vi "initialize hardware.vi"(7 "Reset (False)":bool, 8 "error in (no error)":errorcluster, 9 "devport":string, 10 "Settings":T1={"devport"="", "Position"={"Axis 1"={"Value"=0.0, "Min"=0.0, "Max"=0.0, "StepSize"=0.0, "Tolerance"=0.0, "ValueActual"=0.0}, "Axis 2"={"Value"=0.0, "Min"=0.0, "Max"=0.0, "StepSize"=0.0, "Tolerance"=0.0, "ValueActual"=0.0}, "Axis 3"={"Value"=0.0, "Min"=0.0, "Max"=0.0, "StepSize"=0.0, "Tolerance"=0.0, "ValueActual"=0.0}}, "Power"={"Axis 1"=enum."off", "Axis 2"=enum."off", "Axis 3"=enum."off"}, "Status"={"Axis 1"=enum."Not referenced", "Axis 2"=enum."Not referenced", "Axis 3"=enum."Not referenced"}, "Backlash"={"Axis 1"={"Value"=0.0, "Min"=0.0, "Max"=0.0, "StepSize"=0.0, "Tolerance"=0.0, "ValueActual"=0.0}, "Axis 2"={"Value"=0.0, "Min"=0.0, "Max"=0.0, "StepSize"=0.0, "Tolerance"=0.0, "ValueActual"=0.0}, "Axis 3"={"Value"=0.0, "Min"=0.0, "Max"=0.0, "StepSize"=0.0, "Tolerance"=0.0, "ValueActual"=0.0}}, "Home"={"Axis 1"={"Value"=0.0, "Min"=0.0, "Max"=0.0, "StepSize"=0.0, "Tolerance"=0.0, "ValueActual"=0.0}, "Axis 2"={"Value"=0.0, "Min"=0.0, "Max"=0.0, "StepSize"=0.0, "Tolerance"=0.0, "ValueActual"=0.0}, "Axis 3"={"Value"=0.0, "Min"=0.0, "Max"=0.0, "StepSize"=0.0, "Tolerance"=0.0, "ValueActual"=0.0}}, "MoveToHardLimit"={"Axis 1"=enum."pos", "Axis 2"=enum."pos", "Axis 3"=enum."pos"}, "relativeMove"={"Axis 1neg"=enum."off", "Axis 2neg"=enum."off", "Axis 3neg"=enum."off", "Axis 1pos"=enum."off", "Axis 2pos"=enum."off", "Axis 3pos"=enum."off"}, "stepsize"={"Value"=0.0, "Min"=0.0, "Max"=0.0, "StepSize"=0.0, "Tolerance"=0.0, "ValueActual"=0.0}, "automotoroff"=enum."off", "ResetBeforeMove"=enum."off", "Enable"={"Axis 1"=enum."on", "Axis 2"=enum."on", "Axis 3"=enum."on"}}, 11 "ESP301 in":refnum<class "ESP301.lvclass">) -> (0 "error out":errorcluster, 2 "VISA resource name out":refnum<visa-resource-name>, 3 "ESP301 out":refnum<class "ESP301.lvclass">)   [LabVIEW 2020, in "ESP301.lvclass"]
uses:
  ESP301.lvclass
  ESP301/SettingsTypdef.ctl
  OnOffTypeDef.ctl
  status_TypDef.ctl
  Hardware limit.ctl
  ESP301.lvclass/ESP301.ctl
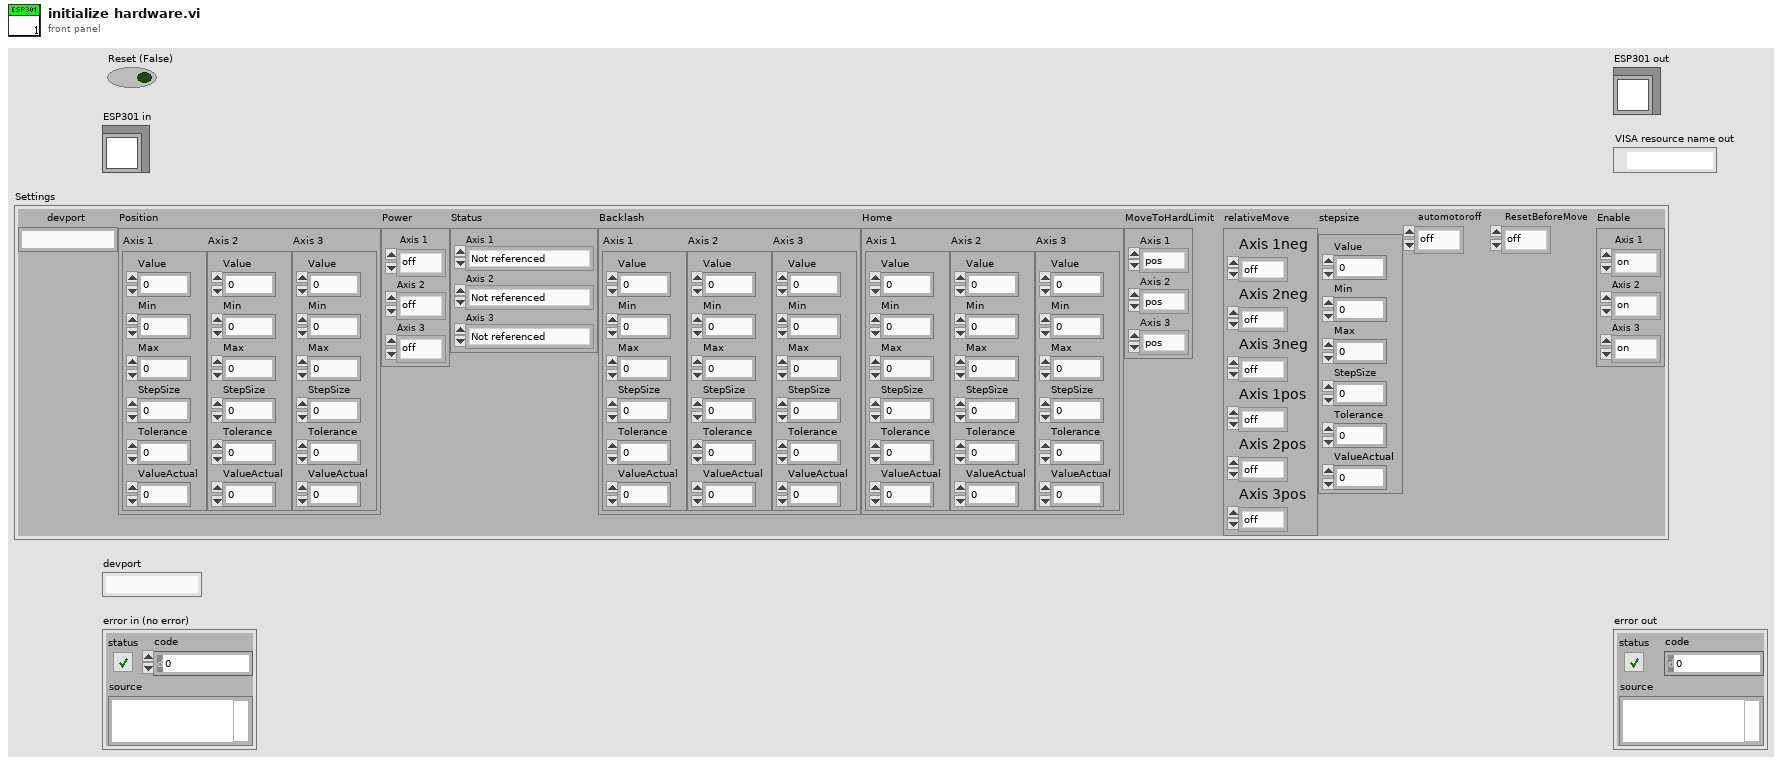
[diagram p1: front panel]
types:
  T1 = typedef "ESP301.lvclass/SettingsTypdef.ctl" = cluster{"devport":string, "Position":cluster{"Axis 1":cluster{"Value":dbl, "Min":dbl, "Max":dbl, "StepSize":dbl, "Tolerance":dbl, "ValueActual":dbl}, "Axis 2":cluster{"Value":dbl, "Min":dbl, "Max":dbl, "StepSize":dbl, "Tolerance":dbl, "ValueActual":dbl}, "Axis 3":cluster{"Value":dbl, "Min":dbl, "Max":dbl, "StepSize":dbl, "Tolerance":dbl, "ValueActual":dbl}}, "Power":cluster{"Axis 1":T2, "Axis 2":T2, "Axis 3":T2}, "Status":cluster{"Axis 1":T3, "Axis 2":T3, "Axis 3":T3}, "Backlash":cluster{"Axis 1":cluster{"Value":dbl, "Min":dbl, "Max":dbl, "StepSize":dbl, "Tolerance":dbl, "ValueActual":dbl}, "Axis 2":cluster{"Value":dbl, "Min":dbl, "Max":dbl, "StepSize":dbl, "Tolerance":dbl, "ValueActual":dbl}, "Axis 3":cluster{"Value":dbl, "Min":dbl, "Max":dbl, "StepSize":dbl, "Tolerance":dbl, "ValueActual":dbl}}, "Home":cluster{"Axis 1":cluster{"Value":dbl, "Min":dbl, "Max":dbl, "StepSize":dbl, "Tolerance":dbl, "ValueActual":dbl}, "Axis 2":cluster{"Value":dbl, "Min":dbl, "Max":dbl, "StepSize":dbl, "Tolerance":dbl, "ValueActual":dbl}, "Axis 3":cluster{"Value":dbl, "Min":dbl, "Max":dbl, "StepSize":dbl, "Tolerance":dbl, "ValueActual":dbl}}, "MoveToHardLimit":cluster{"Axis 1":T4, "Axis 2":T4, "Axis 3":T4}, "relativeMove":cluster{"Axis 1neg":T2, "Axis 2neg":T2, "Axis 3neg":T2, "Axis 1pos":T2, "Axis 2pos":T2, "Axis 3pos":T2}, "stepsize":cluster{"Value":dbl, "Min":dbl, "Max":dbl, "StepSize":dbl, "Tolerance":dbl, "ValueActual":dbl}, "automotoroff":T2, "ResetBeforeMove":T2, "Enable":cluster{"Axis 1":T2, "Axis 2":T2, "Axis 3":T2}}
  T2 = typedef "OnOffTypeDef.ctl" = enum16{"off", "on"}
  T3 = typedef "status_TypDef.ctl" = enum16{"Not referenced", "Homing", "Moving", "Ready"}
  T4 = typedef "Hardware limit.ctl" = enum16{"pos", "neg"}
  T5 = cluster{"Axis 1":cluster{"Value":dbl, "Min":dbl, "Max":dbl, "StepSize":dbl, "Tolerance":dbl, "ValueActual":dbl}, "Axis 2":cluster{"Value":dbl, "Min":dbl, "Max":dbl, "StepSize":dbl, "Tolerance":dbl, "ValueActual":dbl}, "Axis 3":cluster{"Value":dbl, "Min":dbl, "Max":dbl, "StepSize":dbl, "Tolerance":dbl, "ValueActual":dbl}}
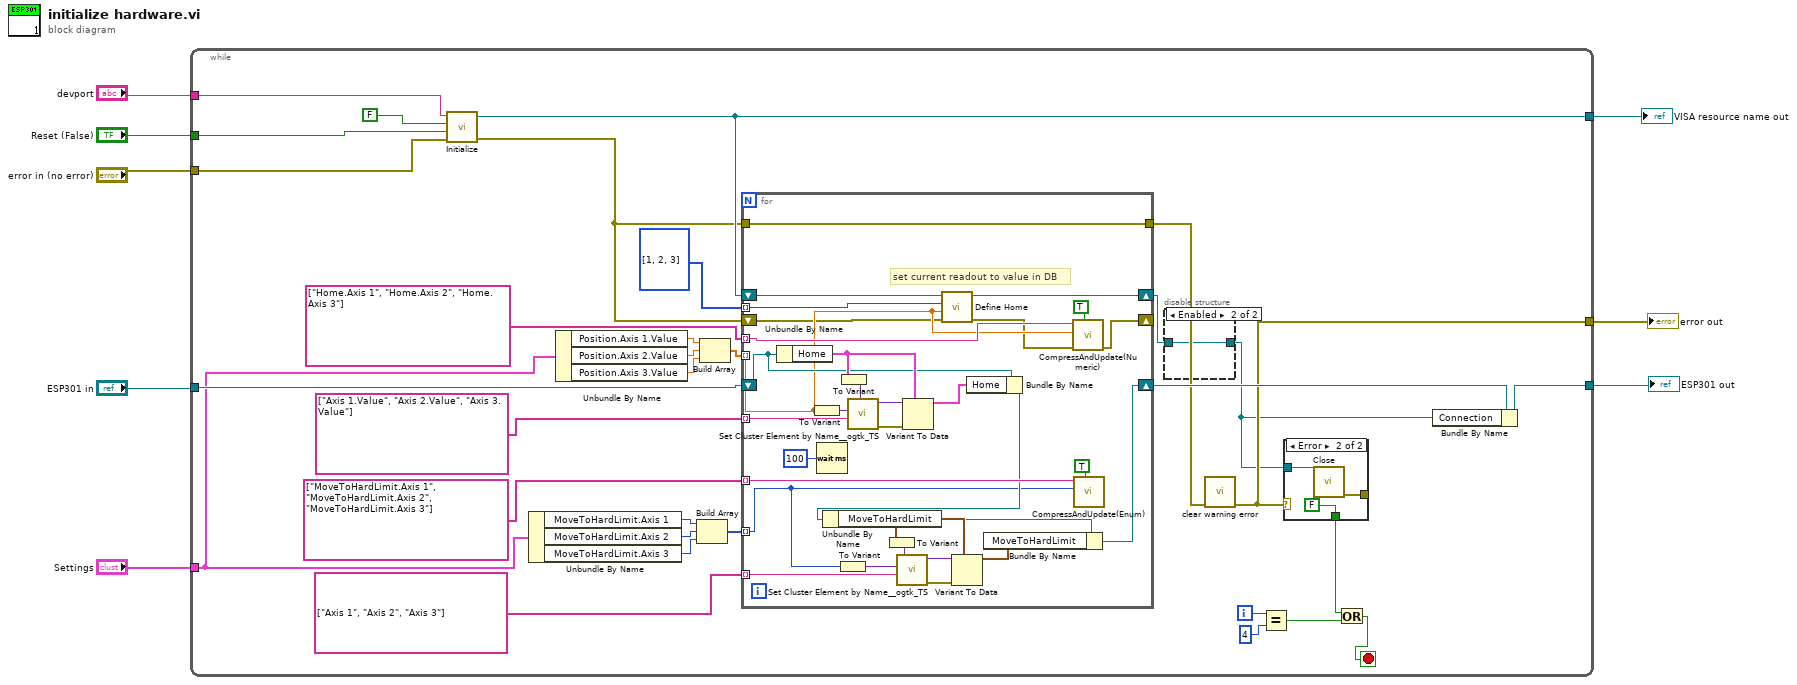
[diagram p0: block diagram]
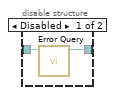
[diagram p2: hidden frame]
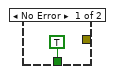
[diagram p3: hidden frame]
diagram:
  n1 = while {
    tunnel: "error in (no error)" -> [w13]
    tunnel: "devport" -> [w16]
    tunnel: "ESP301 in" -> [w35]
    tunnel: [w10] -> w4
    tunnel: [w15] -> w5
    tunnel: "Settings" -> [w24]
    tunnel: [w19] -> w7
    tunnel: "Reset (False)" -> [w11]
    i -> [w23]
    stop <- w20 stop-if-true
    n2 = call "Initialize.vi"("VISA resource name"=w16, "ID Query (True)"=FALSE, "Reset (False)"=w11, "error in (no error)"=w13) -> ("VISA resource name out"=w15:refnum<visa-resource-name>, "error out"=w14:errorcluster)  [unwired: 5 in]
    n3 = Unbundle By Name(w24) -> ("MoveToHardLimit.Axis 1"=w27:T4, "MoveToHardLimit.Axis 2"=w28:T4, "MoveToHardLimit.Axis 3"=w29:T4)
    n4 = Unbundle By Name(w24) -> ("Position.Axis 1.Value"=w39:dbl, "Position.Axis 2.Value"=w38:dbl, "Position.Axis 3.Value"=w37:dbl)
    n5 = Build Array(w27, w28, w29) -> (w26:T4[])
    n6 = Build Array(w39, w38, w37) -> (w36:dbl[])
    n7 = for {
      shift-right: [w69] -> w31
      shift-left: w15 -> [w70]
      tunnel: i32[] [1, 2, 3] -> [w68] mode=indexing
      tunnel: w36 -> [w67] mode=indexing
      shift-right: [w56] -> w34
      shift-left: w35 -> [w74]
      tunnel: string[] ["Axis 1.Value", "Axis 2.Value", "Axis 3.Value"] ("set following Variables (empty = all avriables)") -> [w73] mode=indexing
      tunnel: string[] ["Home.Axis 1", "Home.Axis 2", "Home.Axis 3"] ("set following Variables (empty = all avriables)") -> [w71] mode=indexing
      shift-right: [w64] -> _
      shift-left: w14 -> [w66]
      tunnel: string[] ["MoveToHardLimit.Axis 1", "MoveToHardLimit.Axis 2", "MoveToHardLimit.Axis 3"] ("set following Variables (empty = all avriables)") -> [w62] mode=indexing
      tunnel: w26 -> [w55] mode=indexing
      tunnel: string[] ["Axis 1", "Axis 2", "Axis 3"] ("set following Variables (empty = all avriables)") -> [w54] mode=indexing
      tunnel: w14 -> [w52]
      tunnel: [w52] -> w17
      # "set current readout to value in DB"
      n8 = Unbundle By Name(w74) -> ("Home"=w77:T5)
      n9 = To Variant(anything=w67) -> (Variant=w49:variant)
      n10 = Wait (ms)(milliseconds to wait=u32 100) -> ()  [unwired: 1 out]
      n11 = To Variant(anything=w55) -> (Variant=w50:variant)
      n12 = To Variant(anything=w77) -> (Variant=w48:variant)
      n13 = call "Set Cluster Element by Name__ogtk_TS.vi"("Element Name (\"\": New Element Data Name)"=w73, "New Element Value"=w49, "Cluster"=w48) -> ("error out"=w75:errorcluster, "VCluster out"=w76:variant)  [unwired: 6 in, 1 out]
      n14 = Variant To Data(error in=w75, type=w77, Variant=w76) -> (data=w78:T5)  [unwired: 1 out]
      n15 = call "Define Home.vi"("error in (no error)"=w66, "Home Position (0 units)"=w67, "Axis (1)"=w68, "VISA resource name"=w70) -> ("error out"=w65:errorcluster, "VISA resource name out"=w69:refnum<visa-resource-name>)  [unwired: 2 in]
      n16 = Bundle By Name(cluster=w74, "Home"=w78) -> (w57:refnum<class "ESP301.lvclass">)
      n17 = Unbundle By Name(w57) -> ("MoveToHardLimit"=w59:cluster{"Axis 1":T4, "Axis 2":T4, "Axis 3":T4})
      n18 = To Variant(anything=w59) -> (Variant=w51:variant)
      n19 = call "Set Cluster Element by Name__ogtk_TS.vi"("Element Name (\"\": New Element Data Name)"=w54, "New Element Value"=w50, "Cluster"=w51) -> ("error out"=w61:errorcluster, "VCluster out"=w60:variant)  [unwired: 6 in, 1 out]
      n20 = Variant To Data(error in=w61, type=w59, Variant=w60) -> (data=w58:cluster{"Axis 1":T4, "Axis 2":T4, "Axis 3":T4})  [unwired: 1 out]
      n21 = Bundle By Name(cluster=w57, "MoveToHardLimit"=w58) -> (w56:refnum<class "ESP301.lvclass">)
      n22 = call "CompressAndUpdate(Numeric).vi"("force CVT update (false)"=TRUE ("force CVT update"), "error in"=w65, "Numeric"=w67, "command or variable name"=w71) -> ("error out"=w64:errorcluster)  [unwired: 7 in]
      n23 = call "CompressAndUpdate(Enum).vi"("force CVT update (false)"=TRUE ("force CVT update"), "enum variant"=w55, "command or variable name"=w62) -> ()  [unwired: 8 in, 1 out]
    }
    n24 = disable-structure shown="Enabled" {
      disable-tunnel: w31 -> [w42 w43]
      disable-tunnel: [w41 w43] -> w9
      frame Disabled {
        n25 = call "Error Query.vi"("VISA resource name"=w42) -> ("VISA resource name out"=w41:refnum<visa-resource-name>)  [unwired: 3 in, 3 out]
      }
      frame Enabled {
      }
    }
    n26 = call "clear warning error.vi"("error in"=w17) -> ("error out"=w19:errorcluster)  [unwired: 10 in]
    n27 = Equal?(x=w23, y=4) -> (x = y?=w21:bool)
    n28 = case shown="Error" w19 {
      tunnel: w9 -> [_ w46]
      tunnel: [TRUE FALSE] -> w18
      tunnel: [_ w45] -> _
      frame No Error {
      }
      frame Error {
        n29 = call "Close.vi"("VISA resource name"=w46) -> ("error out"=w45:errorcluster)  [unwired: 10 in]
      }
    }
    n30 = Or(x=w18, y=w21) -> (x .or. y?=w20:bool)
    n31 = Bundle By Name(cluster=w34, "Connection"=w9) -> (w10:refnum<class "ESP301.lvclass">)
  }
  "error out" <- w7
  "VISA resource name out" <- w5
  "ESP301 out" <- w4
